vi "B MeasurementTriton.vi"(7 "error out 2":errorcluster, 10 "VISA resource name 2":refnum<visa-resource-name>) -> (0 "error out":errorcluster, 2 "reading":string, 3 "VISA resource name":refnum<visa-resource-name>, 4 "Measuremet":dbl)   [LabVIEW 2021]
panel:
  out "String":string
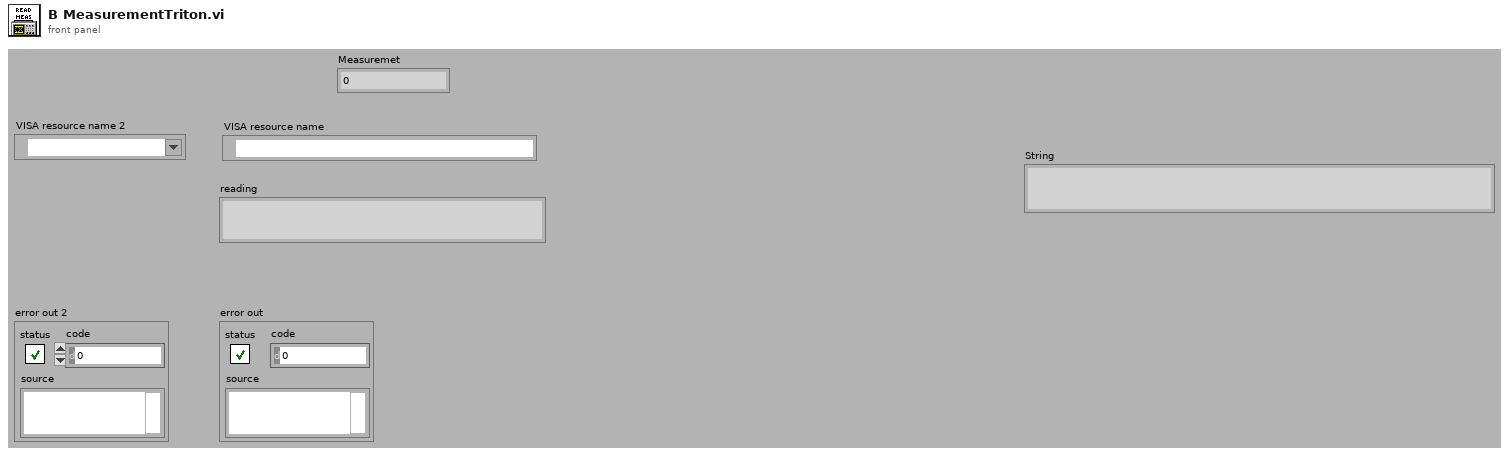
[diagram p1: front panel]
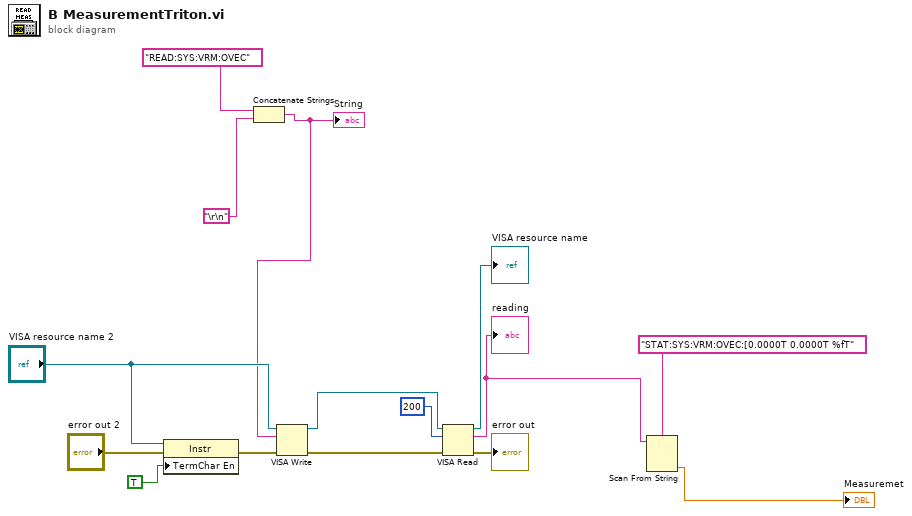
[diagram p0: block diagram]
diagram:
  n1 = property class="Instr"(reference="VISA resource name 2", error in="error out 2", "TermChar En"=TRUE ("Message Based Settings:Termination Character Enable")) -> (error out=w9:errorcluster)  [unwired: 1 out]
  n2 = Concatenate Strings("READ:SYS:VRM:OVEC", "\r\n") -> (w1:string)
  "String" <- w1
  n3 = VISA Write(VISA resource name="VISA resource name 2", write buffer=w1, error in (no error)=w9) -> (VISA resource name out=w13:refnum<visa-resource-name>, error out=w7:errorcluster)  [unwired: 1 out]
  n4 = VISA Read(VISA resource name=w13, byte count=u32 200, error in (no error)=w7) -> (VISA resource name out=→"VISA resource name":refnum<visa-resource-name>, read buffer=w6:string, error out=→"error out":errorcluster)  [unwired: 1 out]
  "reading" <- w6
  n5 = Scan From String(format string="STAT:SYS:VRM:OVEC:[0.0000T 0.0000T %fT", input string=w6) -> (output 1=→"Measuremet":dbl)  [unwired: 3 in, 3 out]
